vi "Execute Channel.vi"(8 "error in (no error)":errorcluster, 9 "Data/Ref":variant, 10 "DAQmx Global Channel":refnum<k21>, 11 "National Instrument USB-6501 in":refnum<class "National Instrument USB-6501.lvclass">) -> (0 "error out":errorcluster, 3 "National Instrument USB-6501 out":refnum<class "National Instrument USB-6501.lvclass">)   [LabVIEW 2016, in "Generic Data Acquisition.lvlib" / "National Instrument USB-6501.lvlib" / "National Instrument USB-6501.lvclass"]
uses:
  National Instrument USB-6501.lvclass
  <vilib>/Utility/Data Type/Type Definitions/Data Type.ctl
  <vilib>/DAQmx/read.llb/DAQmx Read (Digital Bool 1Line 1Point).vi
  <vilib>/DAQmx/write.llb/DAQmx Write (Digital Bool 1Line 1Point).vi
  <vilib>/DAQmx/miscellaneous.llb/DAQmx Fill In Error Info.vi
  <vilib>/Utility/Data Type/NI_Data Type.lvlib
panel:
  out "Type":T1
  out "error out 2":errorcluster
  out "i":i32
  out "x = y?":bool
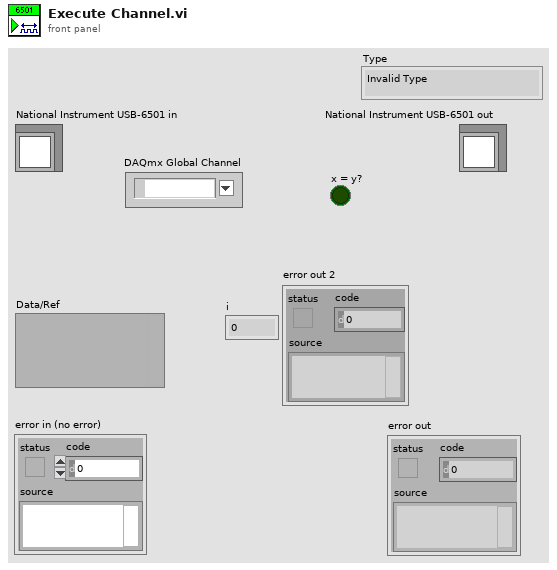
[diagram p1: front panel]
types:
  T1 = typedef "NI_Data Type.lvlib/Data Type.ctl" = enum8{"Invalid Type", "Void", "I8", "I16", "I32", "I64", "U8", "U16", "U32", "U64", "Single Float", "Double Float", "Extended Float", "Single Complex", "Double Complex", "Extended Complex", "Enum U8", "Enum U16", "Enum U32", "Enum U64", "Single Float With Unit", "Double Float With Unit", "Extended Float With Unit", "Single Complex with Unit", "Double Complex with Unit", "Extended Complex with Unit", "Boolean", "String", "Path", "Picture", "Tag", "Array", "Cluster", "Variant", "LV Variant", "Waveform", "Timestamp", "Digital Waveform", "Digital Data", "ExpressData", "Refnum", "External Data", "VI", "Poly VI", "LabVIEW Class Instance", "Fixed Point"}
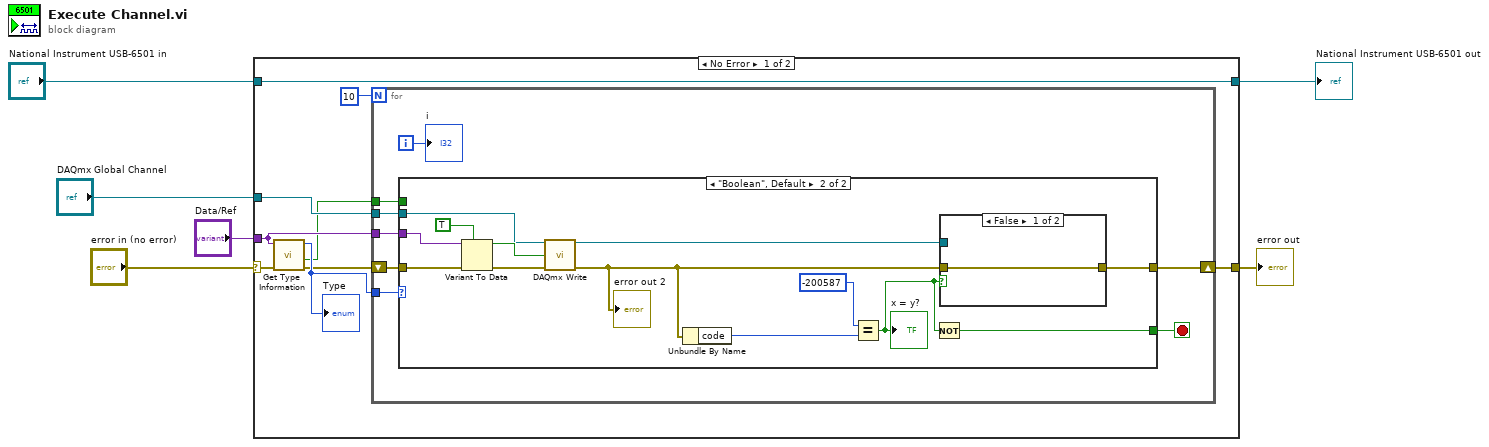
[diagram p0: block diagram]
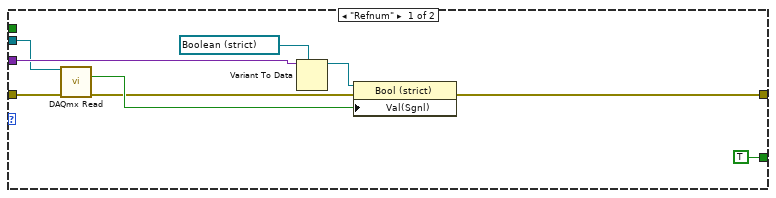
[diagram p2: hidden frame]
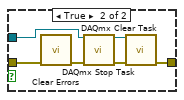
[diagram p3: hidden frame]
diagram:
  n1 = case shown="No Error" "error in (no error)" {
    selector: "error in (no error)" -> [w10 w54]
    tunnel: [w13 w54] -> w5
    tunnel: [w15 w53] -> w3
    tunnel: "National Instrument USB-6501 in" -> [w15 w53]
    tunnel: "Data/Ref" -> [w11 _]
    tunnel: "DAQmx Global Channel" -> [w14 _]
    frame No Error {
      n2 = call <vilib>:"Get Type Information.vi"("error in (no error)"=w10, "Variant"=w11) -> ("error out"=w8:errorcluster, "Type Definition"=w7:bool, "Type"=w9:T1)  [unwired: 5 in, 2 out]
      "Type" <- w9
      n3 = for {
        N: 10 -> [_]
        tunnel: w14 -> [w23]
        tunnel: w9 -> [w20]
        tunnel: w11 -> [w19]
        tunnel: w7 -> [w18]
        shift-right: [w21] -> w13
        shift-left: w8 -> [w22]
        i -> [w16]
        stop <- w17 stop-if-true
        n4 = case shown="\"Boolean\", Default" w20 {
          tunnel: w23 -> [w24 w34]
          tunnel: w22 -> [w25 w35]
          tunnel: [w27 w39] -> w21
          tunnel: w19 -> [w32 w45]
          tunnel: w18 -> [_ _]
          tunnel: [TRUE w41] -> w17
          frame "Refnum" {
            n5 = call-poly <vilib>:"DAQmx Read.vi"("task/channels in"=w24, "error in"=w25) -> ("data"=w29:bool, "error out"=w28:errorcluster)  [unwired: 11 in, 1 out]
            n6 = Variant To Data(type=refnum<vi> refnum ("Bool Refnum"), Variant=w32) -> (data=w30:refnum<vi>)  [unwired: 1 in, 1 out]
            n7 = property class="Bool (strict)"(reference=w30, error in=w28, "Val(Sgnl)"=w29) -> (error out=w27:errorcluster)  [unwired: 1 out]
          }
          frame "Boolean", Default {
            n8 = Variant To Data(error in=w35, type=TRUE, Variant=w45) -> (data=w43:bool, error out=w33:errorcluster)
            n9 = call-poly <vilib>:"DAQmx Write.vi"("task/channels in"=w34, "data"=w43, "error in"=w33) -> ("task out"=w38:refnum<k21>, "error out"=w40:errorcluster)  [unwired: 10 in, 1 out]
            "error out 2" <- w40
            n10 = Unbundle By Name(w40) -> ("code"=w42:i32)
            n11 = Equal?(x=-200587 ("Numeric"), y=w42) -> (x = y?=w36:bool)
            "x = y?" <- w36
            n12 = Not(x=w36) -> (.not. x?=w41:bool)
            n13 = case shown="False" w36 {
              tunnel: w40 -> [w46 w52]
              tunnel: [w46 w47] -> w39
              tunnel: w38 -> [_ w49]
              frame False {
              }
              frame True {
                n14 = call <vilib>:"Clear Errors.vi"("error in (no error)"=w52) -> ("error out"=w51:errorcluster)  [unwired: 5 in, 1 out]
                n15 = call <vilib>:"DAQmx Stop Task.vi"("task/channels in"=w49, "error in"=w51) -> ("task out"=w48:refnum<k21>, "error out"=w50:errorcluster)  [unwired: 12 in]
                n16 = call <vilib>:"DAQmx Clear Task.vi"("task in"=w48, "error in"=w50) -> ("error out"=w47:errorcluster)  [unwired: 13 in]
              }
            }
          }
        }
        "i" <- w16
      }
    }
    frame Error {
    }
  }
  "error out" <- w5
  "National Instrument USB-6501 out" <- w3
